vi "Add to Tree.vi"(7 "Add children? (T)":bool=TRUE, 8 "error in (no error)":errorcluster, 9 "Parent Tag":string, 10 "Tree Manager in":refnum<class "Tree Manager.lvclass">, 11 "Element Array in":refnum<class "Element Array.lvclass">) -> (0 "error out":errorcluster, 2 "Tree Manager out":refnum<class "Tree Manager.lvclass">, 3 "Element Array out":refnum<class "Element Array.lvclass">)   [LabVIEW 2020, in "VILab.lvlib" / "Element Array.lvclass"]
uses:
  Element Array.lvclass
  Tree Manager/Tree Manager.lvclass
  Data Item/Data Item.lvclass
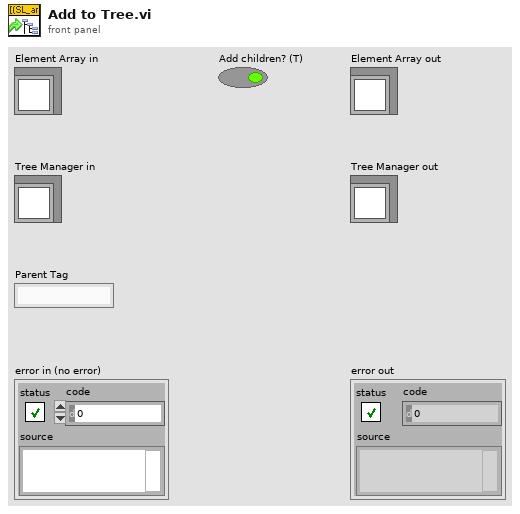
[diagram p1: front panel]
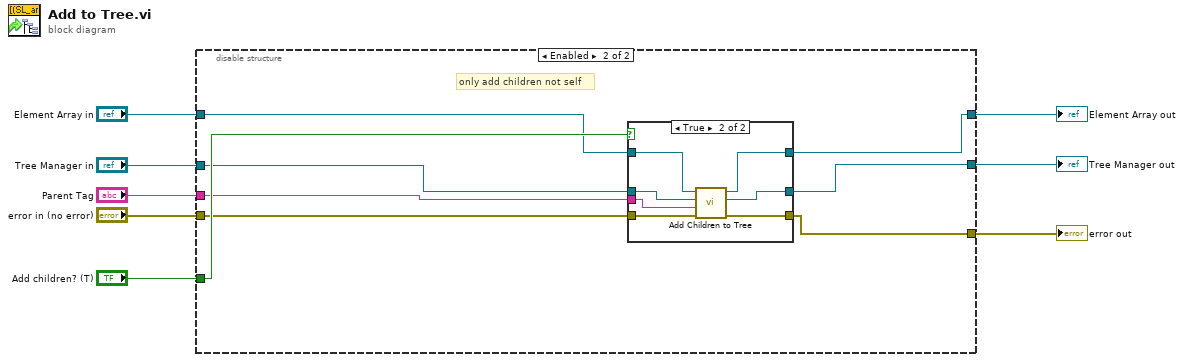
[diagram p0: block diagram]
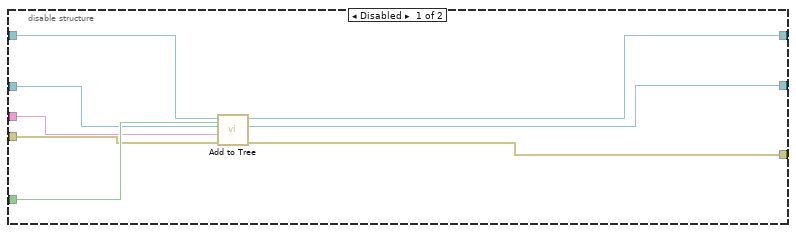
[diagram p2: hidden frame]
diagram:
  n1 = disable-structure shown="Enabled" {
    disable-tunnel: "Add children? (T)" -> [w16 w24]
    disable-tunnel: "Element Array in" -> [w15 w18]
    disable-tunnel: [w14 w19] -> w6
    disable-tunnel: "Parent Tag" -> [w13 w17]
    disable-tunnel: "error in (no error)" -> [w12 w23]
    disable-tunnel: "Tree Manager in" -> [w11 w22]
    disable-tunnel: [w10 w20] -> w7
    disable-tunnel: [w9 w21] -> w8
    frame Disabled {
      n2 = call-parent "Add to Tree.vi"("Add children? (T)"=w16, "error in (no error)"=w12, "Parent Tag"=w13, "Tree Manager in"=w11, "Data Item in"=w15) -> ("error out"=w9:errorcluster, "Tree Manager out"=w10:refnum<class "Tree Manager.lvclass">, "Data Item out"=w14:refnum<class "Element Array.lvclass">)  [unwired: 4 in]
    }
    frame Enabled {
      # "only add children not self"
      n3 = case shown="True" w24 {
        tunnel: w22 -> [w26 w34]
        tunnel: w23 -> [w25 w32]
        tunnel: w17 -> [_ w33]
        tunnel: [w26 w30] -> w20
        tunnel: w18 -> [w27 w28]
        tunnel: [w27 w31] -> w19
        tunnel: [w25 w29] -> w21
        frame False {
        }
        frame True {
          n4 = call-dynamic "Add Children to Tree.vi"("error in (no error)"=w32, "Parent Tag"=w33, "Tree Manager in"=w34, "Element Array in"=w28) -> ("error out"=w29:errorcluster, "Tree Manager out"=w30:refnum<class "Tree Manager.lvclass">, "Element Array out"=w31:refnum<class "Element Array.lvclass">)  [unwired: 5 in]
        }
      }
    }
  }
  "error out" <- w8
  "Element Array out" <- w6
  "Tree Manager out" <- w7
